vi "Swerve Controller.vi"(8 "error in":errorcluster) -> ()   [LabVIEW 2023]
doc: "This VI executes continuously carrying out the current operation and responding to updates or new operations. It will often contain the timing or control code that is difficult to place directly in TeleOp. This VI generally opens all sensors and motors and isolates the rest of the robot code from knowing how the operations are carried out."
uses:
  <vilib>/Rock Robotics/WPI/Framework/Completion Status.ctl
  Swerve Setpoints2.ctl
  Swerve Operations.ctl
  Framework/Robot Global Data.vi
  <vilib>/addons/control/pid/pid.llb/PID (DBL).vi
  <vilib>/addons/control/pid/NI_PID_pid.lvlib
  <vilib>/Rock Robotics/Network Tables/NT Write Boolean.vi
panel:
  out "error out":errorcluster
  out "x-y":u32
  in  "Tape":T1={"proportional gain (Kc)"=1.0, "integral time (Ti, min)"=0.01, "derivative time (Td, min)"=0.0} {"derivative time (Td, min)" format="%.3f"; "integral time (Ti, min)" format="%.3f"; "proportional gain (Kc)" format="%.3f"}
  in  "AprilTag":T1={"proportional gain (Kc)"=1.0, "integral time (Ti, min)"=0.01, "derivative time (Td, min)"=0.0} {"derivative time (Td, min)" format="%.3f"; "integral time (Ti, min)" format="%.3f"; "proportional gain (Kc)" format="%.3f"}
  in  "Look At Cube":T1={"proportional gain (Kc)"=0.001, "integral time (Ti, min)"=0.0, "derivative time (Td, min)"=0.0}
  in  "Look At Cone":T1={"proportional gain (Kc)"=0.004, "integral time (Ti, min)"=0.0, "derivative time (Td, min)"=0.01}
  in  "Balance":T1={"proportional gain (Kc)"=0.011, "integral time (Ti, min)"=0.0, "derivative time (Td, min)"=0.0} {"derivative time (Td, min)" format="%.3f"; "integral time (Ti, min)" format="%.3f"; "proportional gain (Kc)" format="%.3f"}
  in  "Drive to Angle(Distance)":T1={"proportional gain (Kc)"=0.9, "integral time (Ti, min)"=0.0, "derivative time (Td, min)"=0.0} {"derivative time (Td, min)" format="%.3f"; "integral time (Ti, min)" format="%.3f"; "proportional gain (Kc)" format="%.3f"}
  in  "Drive to Angle(Distance)":T1={"proportional gain (Kc)"=0.022, "integral time (Ti, min)"=0.0, "derivative time (Td, min)"=0.0} {"derivative time (Td, min)" format="%.3f"; "integral time (Ti, min)" format="%.3f"; "proportional gain (Kc)" format="%.3f"}
  out "Gyro":dbl
  in  "Drive to angle(Time)":T1={"proportional gain (Kc)"=0.019999999999999574, "integral time (Ti, min)"=0.0, "derivative time (Td, min)"=0.0} {"derivative time (Td, min)" format="%.3f"; "integral time (Ti, min)" format="%.3f"; "proportional gain (Kc)" format="%.3f"}
  in  "Turn to Angle":T1={"proportional gain (Kc)"=0.019999999999999574, "integral time (Ti, min)"=0.0, "derivative time (Td, min)"=0.0} {"derivative time (Td, min)" format="%.3f"; "integral time (Ti, min)" format="%.3f"; "proportional gain (Kc)" format="%.3f"}
  in  "Interactive Values":T2
  out "Current\nCmd":string="Started at  16:27:40.452\nDefault: Reserve,  S 0.0, D 0.000000"
  in  "Buttons":cluster{"Execute Cmd":bool, "Abort Cmd":bool}
  out "Command Timing":cluster{"Start Time (ms)":u32, "Iterations":i32}={"Start Time (ms)"=1585114, "Iterations"=-1}
  out "Status":T4=enum."Aborted"
  # "Tip: It may be helpful to observe inputs and sensor values.\nYou may also want to display tuning or debugging controls."
  # "Interactive Command: You may fill in the settings for a command\nand schedule it with the Execute button. You can observe and abort\nany command while fine tuning the code for the controller."
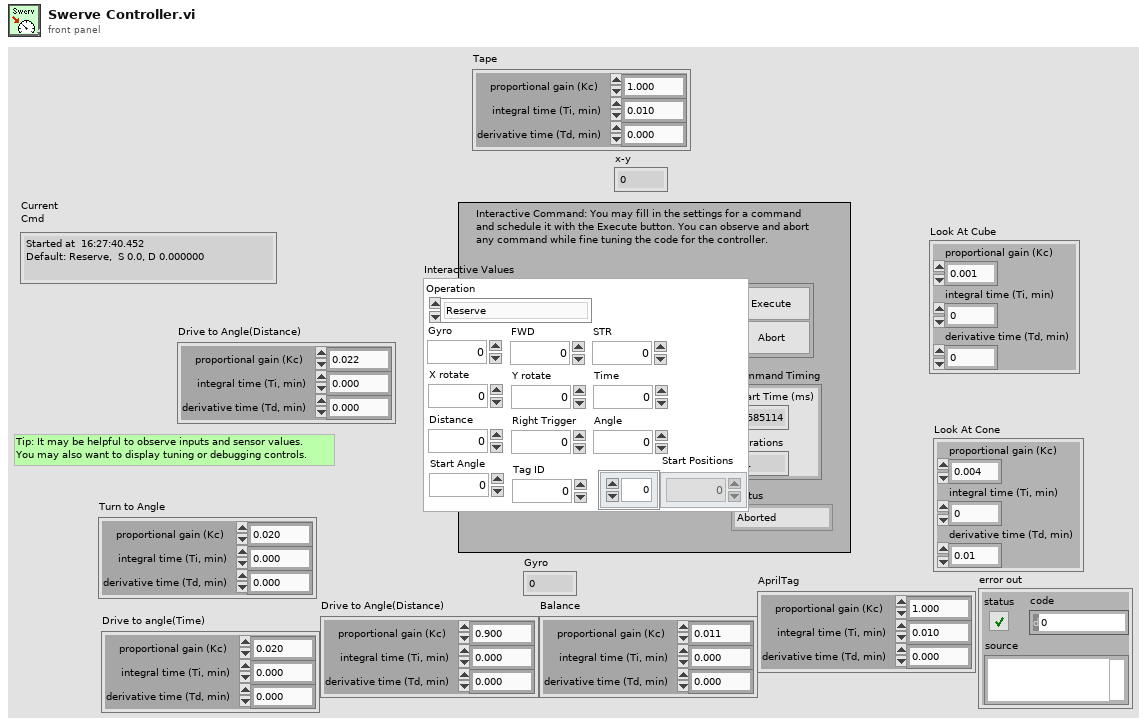
[diagram p1: front panel]
types:
  T1 = cluster{"proportional gain (Kc)":dbl, "integral time (Ti, min)":dbl, "derivative time (Td, min)":dbl}
  T2 = typedef "Swerve Setpoints2.ctl" = cluster{"Operation":T3, "Gyro":dbl, "FWD":dbl, "STR":dbl, "X rotate":dbl, "Y rotate":dbl, "Time":dbl, "Distance":dbl, "Right Trigger":dbl, "Angle":dbl, "Start Angle":dbl, "Tag ID":dbl, "Start Positions":dbl[]}
  T3 = typedef "Swerve Operations.ctl" = enum16{"Reserve", "Read Current", "Immediate", "Stop", "Balance", "Direct  Joystick Drive", "Joystick Drive", "Drive for Distance", "Drive for Time", "Turn to Angle", "Drive to Angle(Time)", "Drive to Angle(Distance)", "Look At Cone", "Look At Cube", "Move To Tape", "Move To Tag"}
  T4 = typedef "Completion Status.ctl" = enum16{"Successful", "Aborted", "Incomplete"}
  T5 = typedef "Command Status Info.ctl" = cluster{"Name":string, "Status":T4, "notifier out":T6}
  T6 = typedef "Completion Notifier.ctl" = refnum<notifier>
  T7 = cluster{"Current Command":T2, "Command Timing":cluster{"Start Time (ms)":u32, "Iterations":i32}, "Command Arguments":cluster{"Command Info":T5, "Description":string, "Default Command":T2, "queue out":refnum<queue>, "Subsystem Name":string}}
  T8 = enum16{"AprilTag", "Reflective Tape", "Custom", "Cube", "Cone"}
  T9 = typedef "ADIS16470 Device Reference.ctl" = cluster{"DevStatus":errorcluster, "Hardware Config":T10, "Calibration Complete":refnum<notifier>, "Status Reference":refnum<data-value>, "Data Reference":refnum<data-value>, "Sychronous Process VI":T14, "Cmd FIFO":refnum<k33>, "Source":T15, "Data FIFO":refnum<k33>, "Calibration Time (ms)":u32, "Data Reference":refnum<data-value>}
  T10 = typedef "ADIS16470 Hardware Configuration.ctl" = cluster{"SPI Clock Rate (Hz)":dbl, "IMU SPI Mode (3)":T11, "IMU Reset Pin":T12, "IMU SPI Bus":T13, "IMU Data Ready Pin":T12, "Stall Config":cluster{"Pow2BytesPerRead":u8, "StallTicks":u16, "CsToSclkTicks":u8}}
  T11 = typedef "WPI_SPIMode.ctl" = enum16{"Mode 0 (Clk Idle Low,Sample on Leading)", "Mode 1 (Clk Idle Low,Sample on Trailing)", "Mode 2 (Clk Idle High,Sample on Leading)", "Mode 3 (Clk Idle High,Sample on Trailing)"}
  T12 = typedef "FPGA_DIOChannel.ctl" = enum8{"DIO 0", "DIO 1", "DIO 2", "DIO 3", "DIO 4", "DIO 5", "DIO 6", "DIO 7", "DIO 8", "DIO 9", "DIO MXP 0", "DIO MXP 1", "DIO MXP 2", "DIO MXP 3", "DIO MXP 4", "DIO MXP 5", "DIO MXP 6", "DIO MXP 7", "DIO MXP 8", "DIO MXP 9", "DIO MXP 10", "DIO MXP 11", "DIO MXP 12", "DIO MXP 13", "DIO MXP 14", "DIO MXP 15", "SPI Port CS1", "SPI Port CS2", "SPI Port CS3", "SPI Port MISO", "SPI Port MOSI", "Invalid"}
  T13 = typedef "spi_bus.ctl" = enum16{"SPI On-Board, CS0", "SPI On-Board, CS1", "SPI On-Board, CS2", "SPI On-Board, CS3", "SPI MXP", "Invalid"}
  T14 = typedef "ADIS16470 Process.ctl" = refnum<vi>
  T15 = typedef "FPGA_CounterEncoderSourceConvertionLVSourceType.ctl" = cluster{"DevStatus":errorcluster, "AnalogTriggerMode?":bool, "DigitalMode":cluster{"DIO Channel":T16}, "AnalogTriggerMode":cluster{"AnalogTriggerIndex":T17, "OutputType":T18}}
  T16 = typedef "FPGA_DIODigitalSourceChannel.ctl" = enum8{"DIO 0", "DIO 1", "DIO 2", "DIO 3", "DIO 4", "DIO 5", "DIO 6", "DIO 7", "DIO 8", "DIO 9", "DIO MXP 0", "DIO MXP 1", "DIO MXP 2", "DIO MXP 3", "DIO MXP 4", "DIO MXP 5", "DIO MXP 6", "DIO MXP 7", "DIO MXP 8", "DIO MXP 9", "DIO MXP 10", "DIO MXP 11", "DIO MXP 12", "DIO MXP 13", "DIO MXP 14", "DIO MXP 15", "SPI Port CS1", "SPI Port CS2", "SPI Port CS3", "SPI Port MISO", "SPI Port MOSI", "Disabled"}
  T17 = typedef "FPGA_AnalogTriggerIndex.ctl" = enum8{"Trig 0", "Trig 1", "Trig 2", "Trig 3", "Trig 4", "Trig 5", "Trig 6", "Trig 7", "Invalid"}
  T18 = typedef "FPGA_AnalogTriggerOutType.ctl" = enum16{"InWindow", "TriggerState", "Rising", "Falling"}
  T19 = typedef "ADIS16470 Data.ctl" = cluster{"XAngle":dbl, "YAngle":dbl, "ZAngle":dbl}
  T20 = typedef "WPI_MotorControlDeviceRef.ctl" = cluster{"DeviceStatus":errorcluster, "Type":T21, "PWM":cluster{"PWM Channel":T22, "DeadBand":T23}, "CAN":cluster{"Device Number":u8, "SetOutput VI Ref":variant, "GetOutput VI Ref":variant, "Enable VI Ref":variant, "Disable VI Ref":variant, "Data":variant}, "Invert":bool, "DIO PWM":cluster{"PWM \"Enable\" Channel":T22, "DIOChannel":T12, "PWM Rate":dbl}}
  T21 = typedef "WPI_MotorControlType.ctl" = enum16{"PWM", "CAN", "DIO PWM"}
  T22 = typedef "FPGA_DIOPWMChannel.ctl" = enum8{"PWM 0", "PWM 1", "PWM 2", "PWM 3", "PWM 4", "PWM 5", "PWM 6", "PWM 7", "PWM 8", "PWM 9", "PWM MXP 0", "PWM MXP 1", "PWM MXP 2", "PWM MXP 3", "PWM MXP 4", "PWM MXP 5", "PWM MXP 6", "PWM MXP 7", "PWM MXP 8", "PWM MXP 9", "Invalid"}
  T23 = typedef "WPI_PWMDeadband.ctl" = cluster{"Name":string, "maxPositivePwm":i32, "minPositivePwm":i32, "centerPwm":i32, "maxNegativePwm":i32, "minNegativePwm":i32, "angularRange":u16}
  T24 = cluster{"tag ID":i32, "Center":cluster{"X":dbl, "Y":dbl}, "homography matrix":dbl[], "decision margin":dbl, "Hamming Dist":i32, "corner points":cluster{"X":dbl, "Y":dbl}[], "Tag Family":string}[]
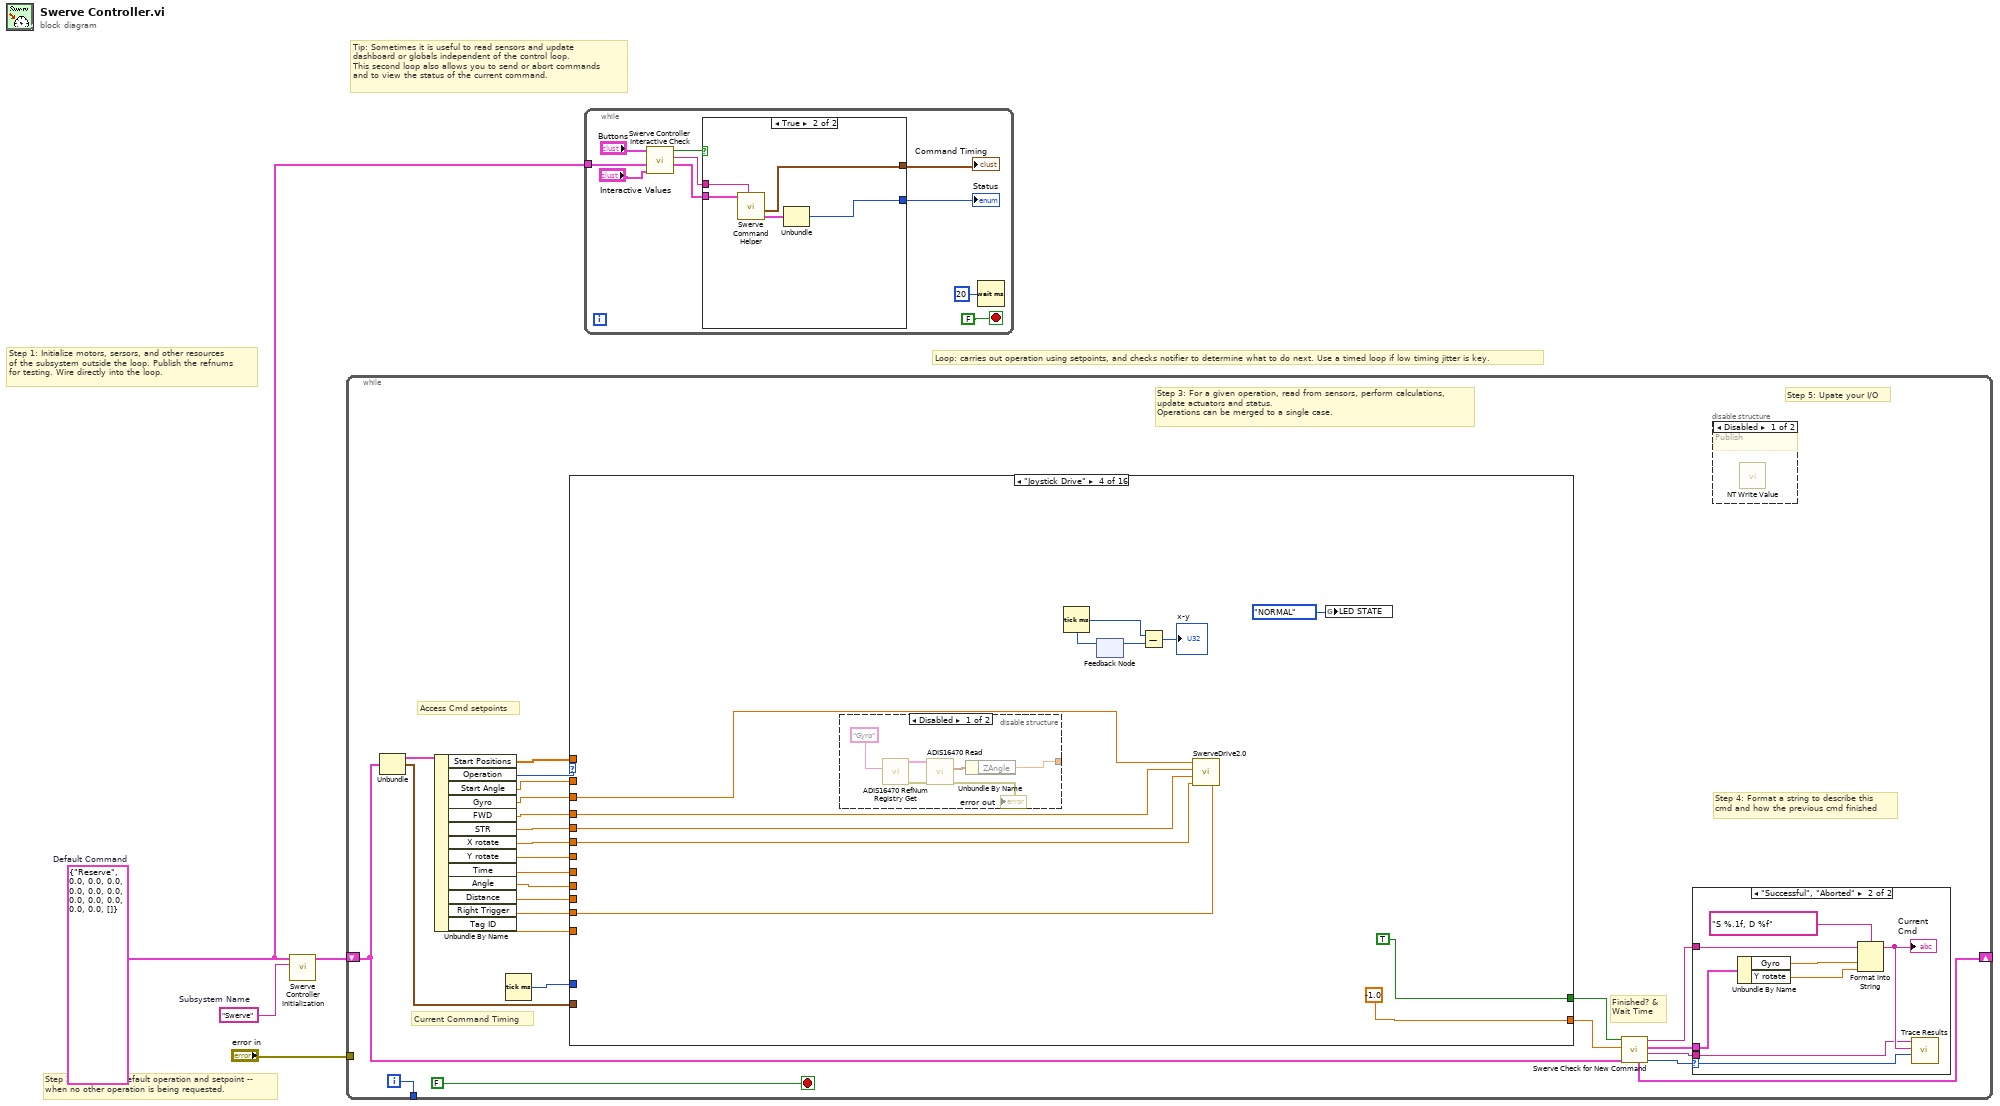
[diagram p0: block diagram]
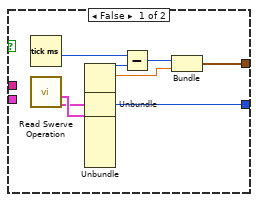
[diagram p2: hidden frame]
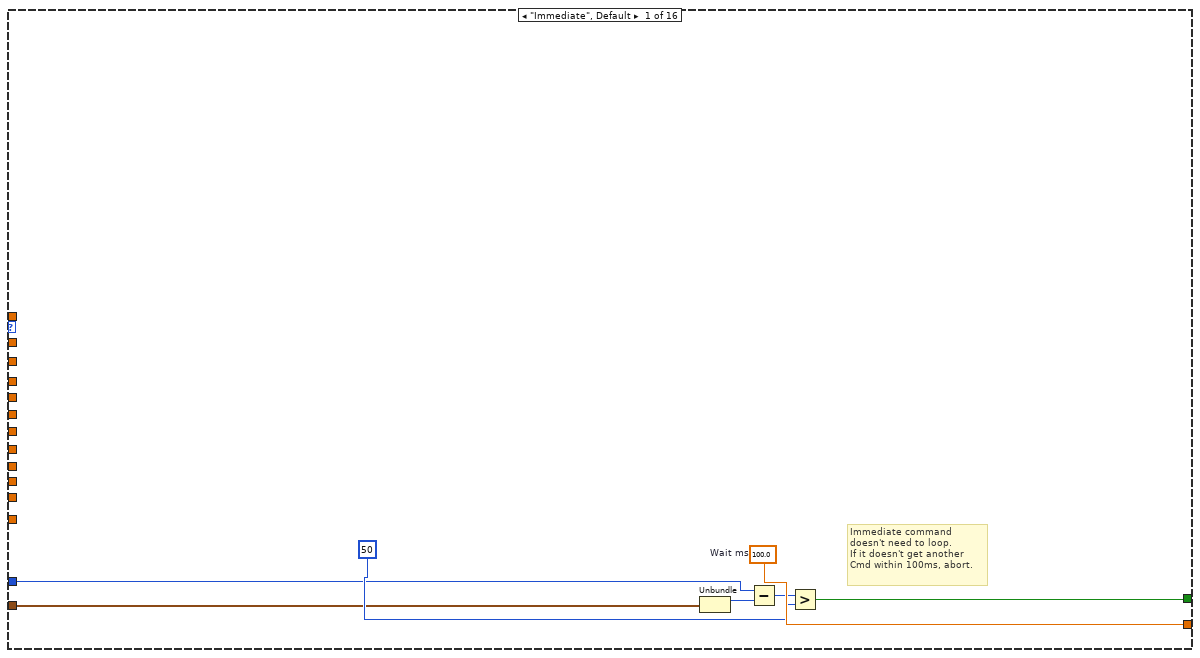
[diagram p3: hidden frame]
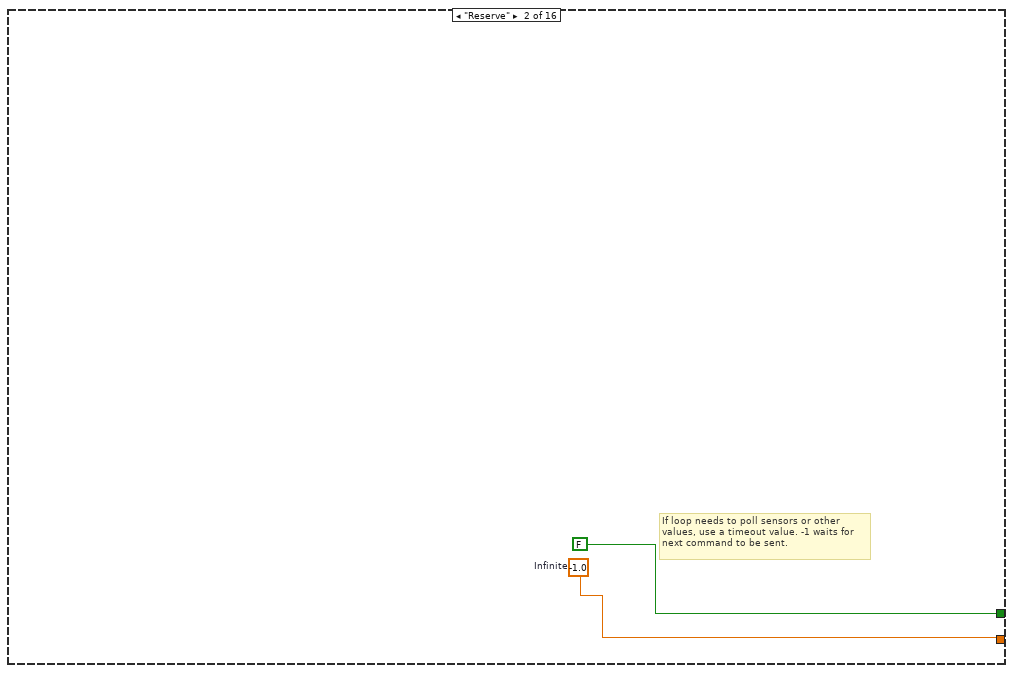
[diagram p4: hidden frame]
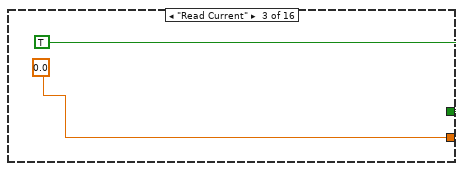
[diagram p5: hidden frame]
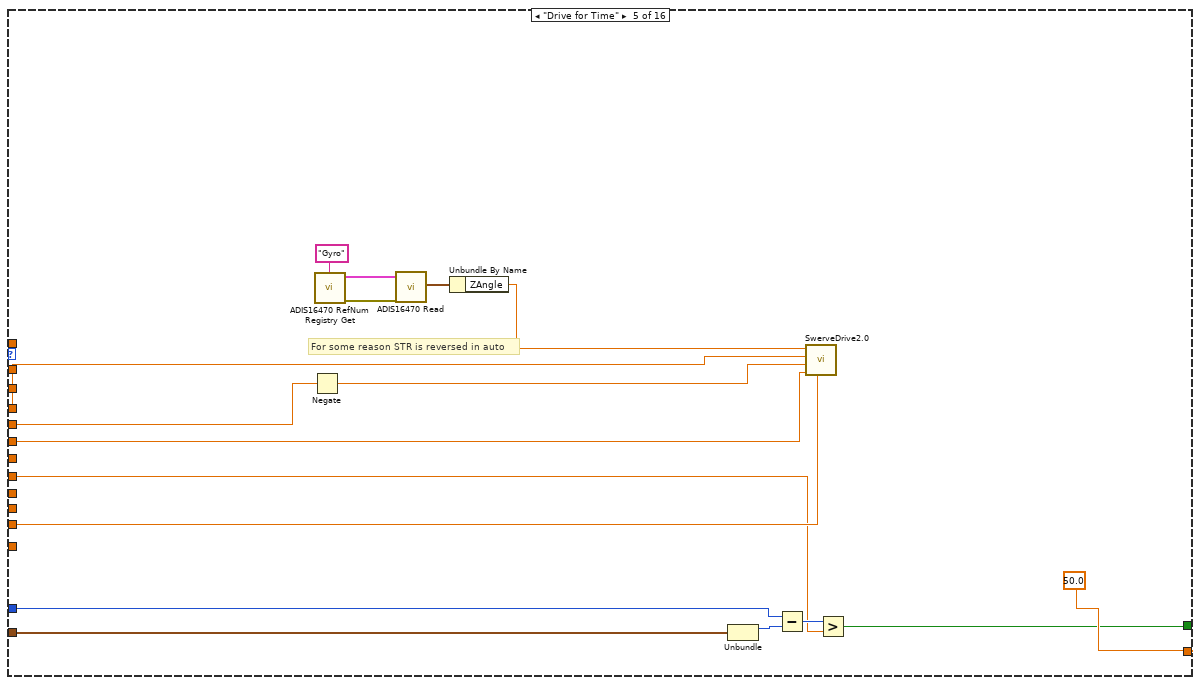
[diagram p7: hidden frame]
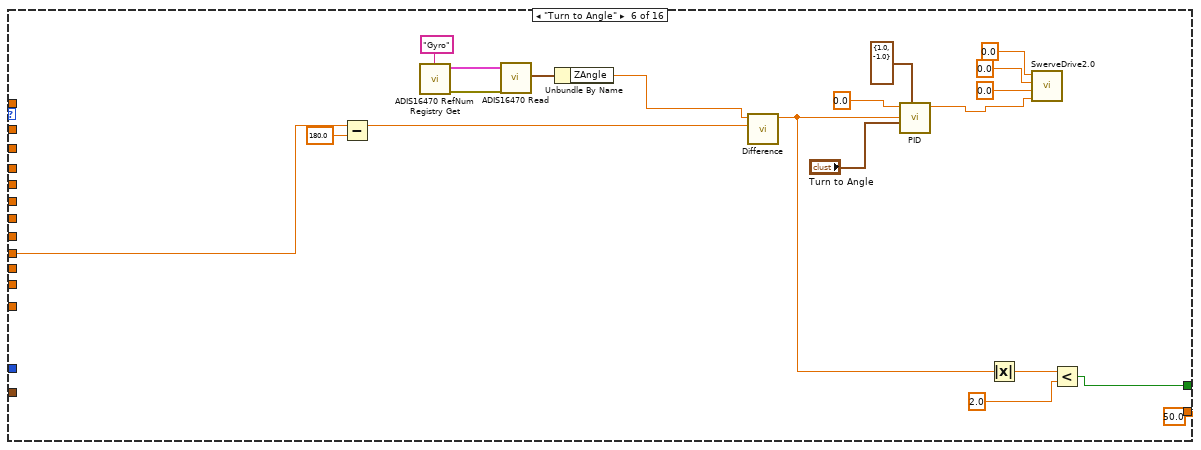
[diagram p8: hidden frame]
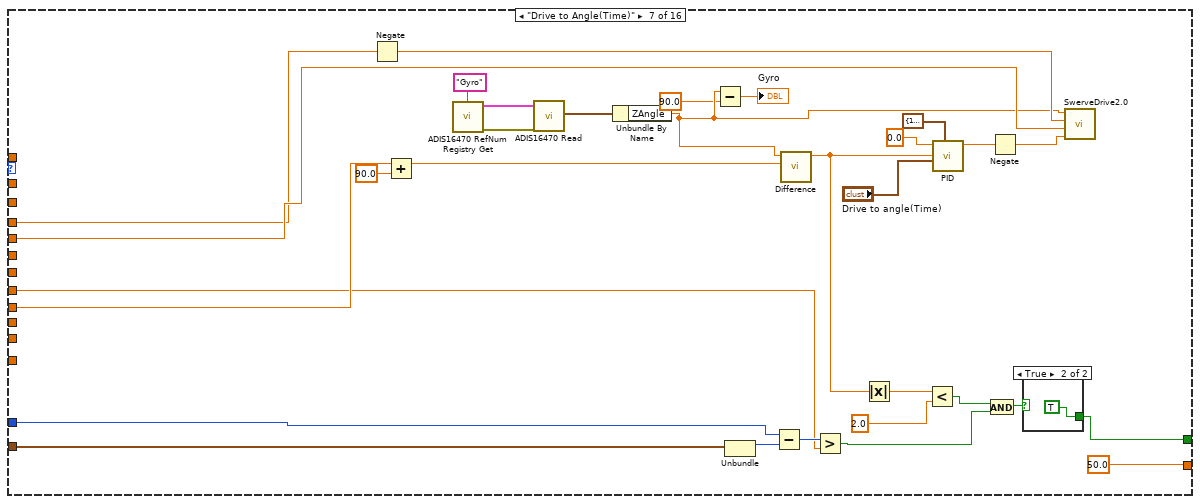
[diagram p9: hidden frame]
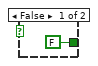
[diagram p10: hidden frame]
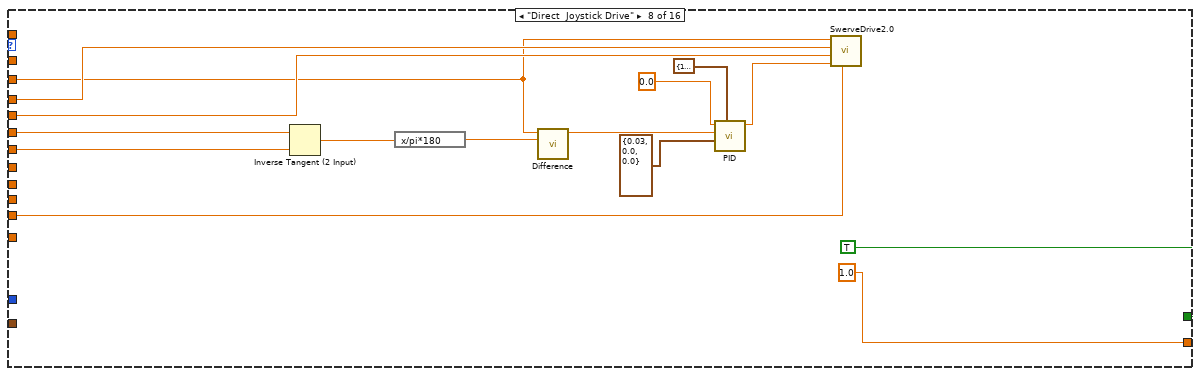
[diagram p11: hidden frame]
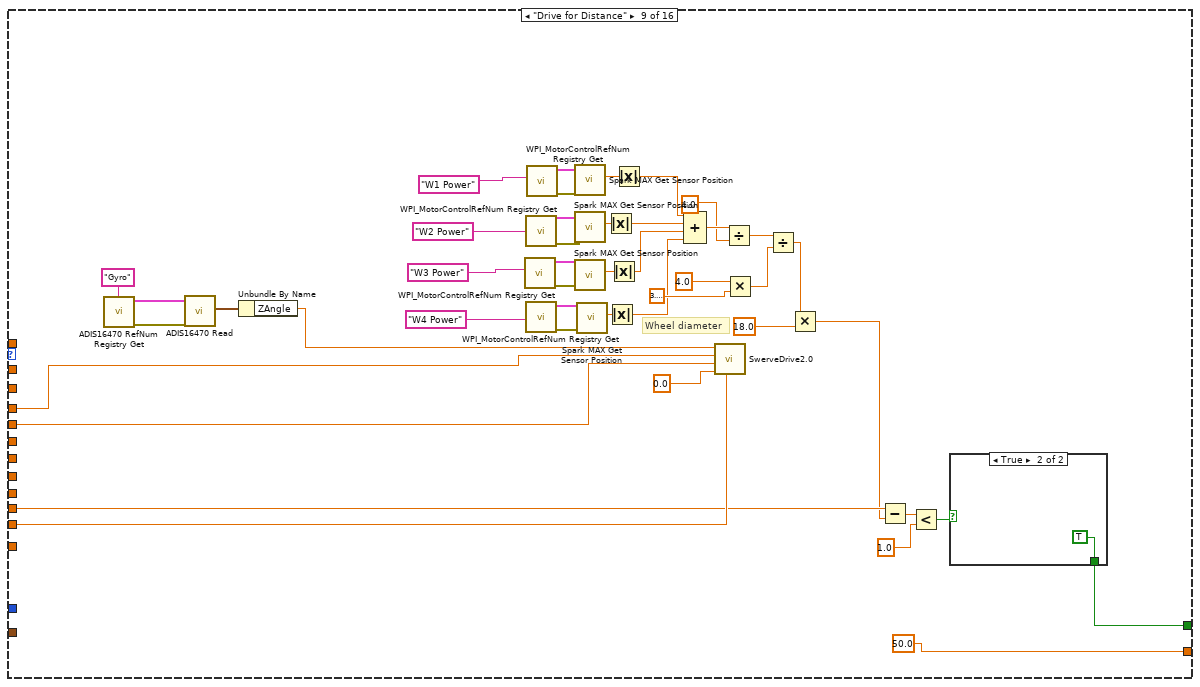
[diagram p12: hidden frame]
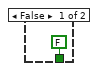
[diagram p13: hidden frame]
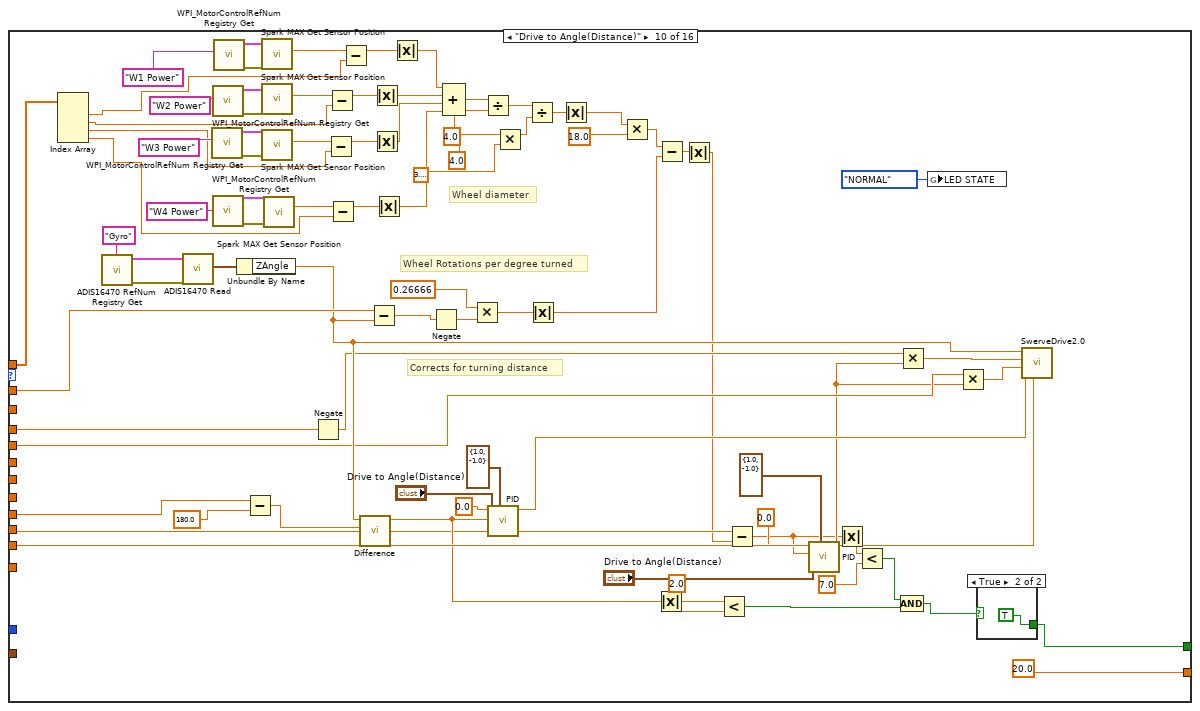
[diagram p14: hidden frame]
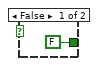
[diagram p15: hidden frame]
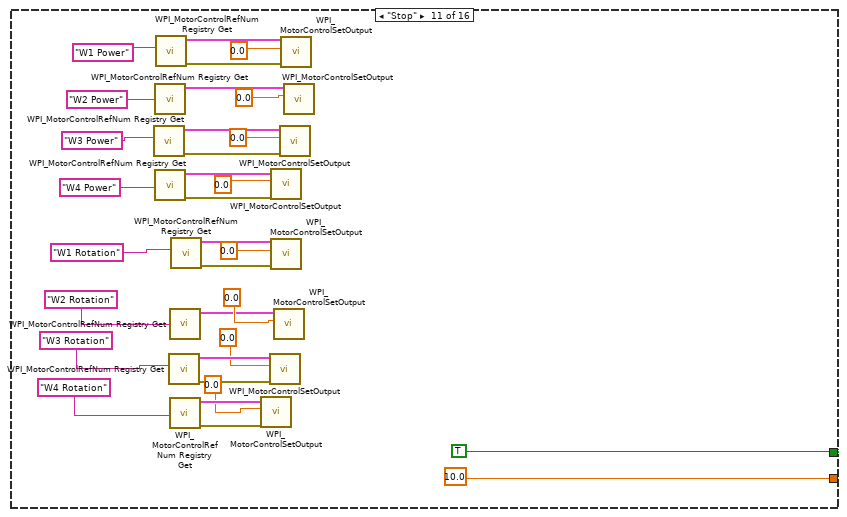
[diagram p16: hidden frame]
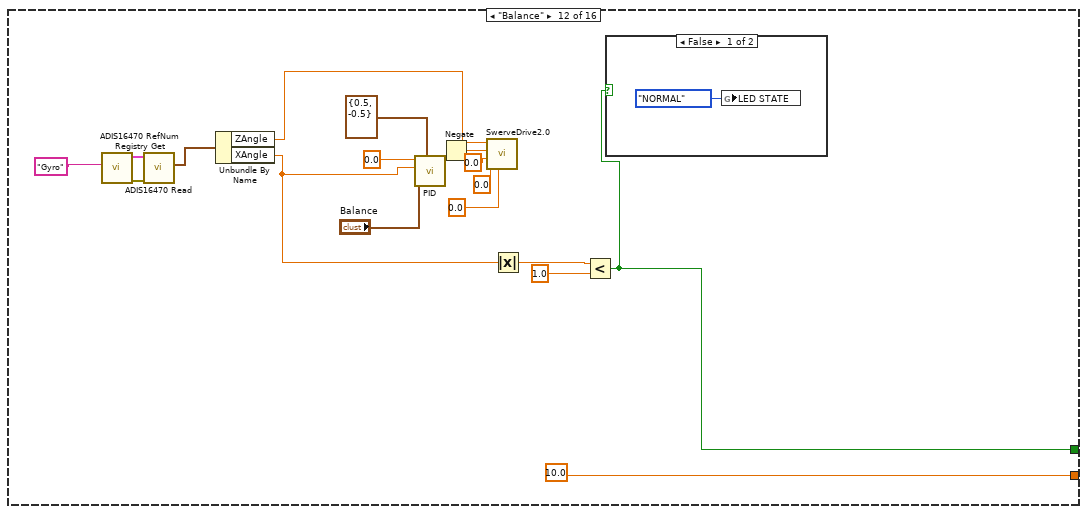
[diagram p17: hidden frame]
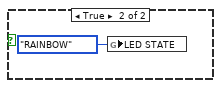
[diagram p18: hidden frame]
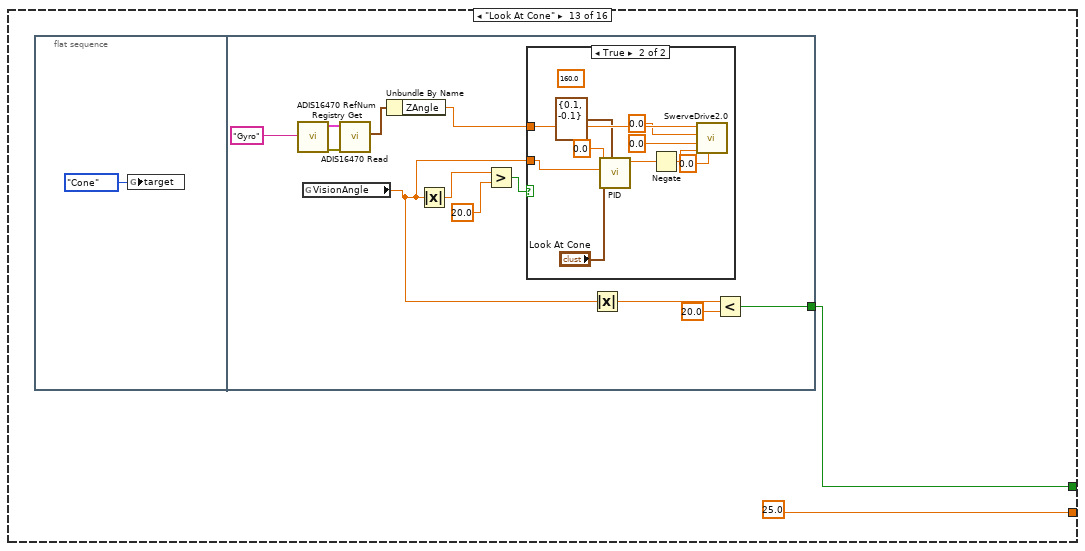
[diagram p19: hidden frame]
diagram:
  w1 = T2 {"Operation"=enum."Reserve", "Gyro"=0.0, "FWD"=0.0, "STR"=0.0, "X rotate"=0.0, "Y rotate"=0.0, "Time"=0.0, "Distance"=0.0, "Right Trigger"=0.0, "Angle"=0.0, "Start Angle"=0.0, "Tag ID"=0.0, "Start Positions"=[]}  # Default Command
  w2 = "Swerve"  # Subsystem Name
  # "Tip: Sometimes it is useful to read sensors and update\ndashboard or globals independent of the control loop.\nThis second loop also allows you to send or abort commands\nand to view the status of the current command."
  # "Step 2: Define the default operation and setpoint --\nwhen no other operation is being requested."
  # "Step 1: Initialize motors, sersors, and other resources\nof the subsystem outside the loop. Publish the refnums\nfor testing. Wire directly into the loop."
  # "Loop: carries out operation using setpoints, and checks notifier to determine what to do next. Use a timed loop if low timing jitter is key."
  n1 = call "Swerve Controller Initialization.vi"("Subsystem Name"=w2, "Default Command"=w1) -> ("Current Command"=w3:T7)  [unwired: 9 in]
  n2 = while {
    shift-right: [w24] -> _
    shift-left: w3 -> [w18]
    tunnel: [w29] -> _
    tunnel: "error in" -> [_]
    i -> [w29]
    stop <- FALSE stop-if-true
    # "Step 5: Upate your I/O"
    # "Step 4: Format a string to describe this\ncmd and how the previous cmd finished"
    # "Current Command Timing"
    # "Access Cmd setpoints"
    # "Finished? &\nWait Time"
    # "Step 3: For a given operation, read from sensors, perform calculations,\nupdate actuators and status.\nOperations can be merged to a single case."
    n3 = Unbundle(w18) -> ("Current Command"=w28:T2, "Command Timing"=w25:cluster{"Start Time (ms)":u32, "Iterations":i32})  [unwired: 1 out]
    n4 = Unbundle By Name(w28) -> ("Start Positions"=w5:dbl[], "Operation"=w27:T3, "Start Angle"=w8:dbl, "Gyro"=w17:dbl, "FWD"=w16:dbl, "STR"=w15:dbl, "X rotate"=w14:dbl, "Y rotate"=w9:dbl, "Time"=w10:dbl, "Angle"=w13:dbl, "Distance"=w12:dbl, "Right Trigger"=w11:dbl, "Tag ID"=w7:dbl)
    n5 = Tick Count (ms)() -> (millisecond timer value=w26:u32)
    n6 = case shown="\"Joystick Drive\"" w27 {
      tunnel: [w37 w39 0.0 ("Time") -1.0 ("Infinite") 50.0 ("Time") 50.0 ("Time") 50.0 ("Time") 1.0 ("Time") 50.0 ("Time") 20.0 ("Time") 10.0 ("Time") 10.0 ("Time") 25.0 ("Time") 25.0 ("Time") 10.0 ("Time") 10.0 ("Time")] -> w23
      tunnel: w25 -> [w33 _ _ _ w69 _ w124 _ _ _ _ _ _ _ _ _]
      tunnel: w26 -> [w32 _ _ _ w70 _ w123 _ _ _ _ _ _ _ _ _]
      tunnel: w17 -> [_ _ _ w42 _ _ _ w130 _ _ _ _ _ _ _ _]
      tunnel: w16 -> [_ _ _ w52 w73 _ w103 w141 w145 w268 _ _ _ _ _ _]
      tunnel: w15 -> [_ _ _ w49 w74 _ w104 w142 w167 w205 _ _ _ _ _ _]
      tunnel: w14 -> [_ _ _ w48 w66 _ _ w136 _ _ _ _ _ _ _ _]
      tunnel: w13 -> [_ _ _ _ _ w80 w102 _ _ w267 _ _ _ _ _ _]
      tunnel: w12 -> [_ _ _ _ _ _ _ _ w165 w221 _ _ _ _ _ _]
      tunnel: w11 -> [_ _ _ w51 w75 _ _ w143 w187 w269 _ _ _ _ _ _]
      tunnel: w10 -> [_ _ _ _ w67 _ w101 _ _ _ _ _ _ _ _ _]
      tunnel: w9 -> [_ _ _ _ _ _ _ w135 _ _ _ _ _ _ _ _]
      tunnel: w8 -> [_ _ _ _ _ _ _ _ _ w217 _ _ _ _ _ _]
      tunnel: w7 -> [_ _ _ _ _ _ _ _ _ _ _ _ _ _ w380 _]
      tunnel: [w31 FALSE ("ignore previous (F)") TRUE ("ignore previous (F)") TRUE ("ignore previous (F)") w59 w76 w96 TRUE ("ignore previous (F)") w144 w203 TRUE ("ignore previous (F)") w306 w326 w351 w379 w415] -> w6
      tunnel: w5 -> [_ _ _ _ _ _ _ _ _ w196 _ _ _ _ _ _]
      frame "Immediate", Default {
        w37 = 100.0  # Wait ms
        # "Immediate command\ndoesn't need to loop.\nIf it doesn't get another\nCmd within 100ms, abort."
        n7 = Unbundle(w33) -> ("Start Time (ms)"=w36:u32)  [unwired: 1 out]
        n8 = Subtract(x=w32, y=w36) -> (x-y=w35:u32)
        n9 = Greater?(x=w35, y=u8 50 ("Left Motor")) -> (0:w31:bool)
      }
      frame "Reserve" {
        w39 = -1.0  # Infinite
        # "If loop needs to poll sensors or other\nvalues, use a timeout value. -1 waits for\nnext command to be sent."
      }
      frame "Read Current" {
      }
      frame "Joystick Drive" {
        n10 = disable-structure shown="Disabled" {
          disable-tunnel: [w54 _] -> _
          frame Disabled {
            n11 = call <vilib>:"ADIS16470 RefNum Registry Get.vi"("refnum name"="Gyro") -> ("error out"=w58:errorcluster, "ADIS16470DevRef out"=w57:T9)  [unwired: 9 in]
            n12 = call <vilib>:"ADIS16470 Read.vi"("error in (no error)"=w58, "ADIS16470DevRef"=w57) -> ("error out"=→"error out":errorcluster, "ADIS16470 Value"=w55:T19)  [unwired: 6 in, 2 out]
            n13 = Unbundle By Name(w55) -> ("ZAngle"=w54:dbl)
          }
          frame Enabled {
          }
        }
        n14 = Tick Count (ms)() -> (millisecond timer value=w46:u32)
        n15 = feedback-in #1(w46) -> ()
        n16 = feedback #1() -> (w45:u32)  [unwired: 1 in]
        n17 = Subtract(x=w46, y=w45) -> (x-y=→"x-y":u32)
        n18 = call "SwerveDrive2.0.vi"("Right Trigger"=w51, "RCW"=w48, "STR"=w49, "FWD"=w52, "Gyro"=w42) -> ()  [unwired: 7 in]
        n19 = global write "Robot Global Data.vi" "LED STATE"(enum16{"NORMAL", "RAINBOW"}."NORMAL" ("LED STATE")) -> ()
      }
      frame "Drive for Time" {
        # "For some reason STR is reversed in auto"
        n20 = Negate(x=w74) -> (-x=w60:dbl)
        n21 = call <vilib>:"ADIS16470 RefNum Registry Get.vi"("refnum name"="Gyro") -> ("error out"=w65:errorcluster, "ADIS16470DevRef out"=w64:T9)  [unwired: 9 in]
        n22 = call <vilib>:"ADIS16470 Read.vi"("error in (no error)"=w65, "ADIS16470DevRef"=w64) -> ("ADIS16470 Value"=w63:T19)  [unwired: 6 in, 3 out]
        n23 = Unbundle By Name(w63) -> ("ZAngle"=w61:dbl)
        n24 = Unbundle(w69) -> ("Start Time (ms)"=w72:u32)  [unwired: 1 out]
        n25 = Subtract(x=w70, y=w72) -> (x-y=w71:u32)
        n26 = call "SwerveDrive2.0.vi"("Right Trigger"=w75, "RCW"=w66, "STR"=w60, "FWD"=w73, "Gyro"=w61) -> ()  [unwired: 7 in]
        n27 = Greater?(x=w71, y=w67) -> (0:w59:bool)
      }
      frame "Turn to Angle" {
        n28 = Subtract(x=w80, y=180.0) -> (x-y=w79:dbl)
        n29 = call <vilib>:"ADIS16470 RefNum Registry Get.vi"("refnum name"="Gyro") -> ("error out"=w90:errorcluster, "ADIS16470DevRef out"=w89:T9)  [unwired: 9 in]
        n30 = call <vilib>:"ADIS16470 Read.vi"("error in (no error)"=w90, "ADIS16470DevRef"=w89) -> ("ADIS16470 Value"=w88:T19)  [unwired: 6 in, 3 out]
        n31 = Unbundle By Name(w88) -> ("ZAngle"=w86:dbl)
        n32 = call "Difference.vi"("Angle"=w79, "Gyro"=w86) -> ("Difference"=w84:dbl)  [unwired: 9 in]
        n33 = call-poly <vilib>:"PID.vi"("output range"=cluster{"output high":dbl, "output low":dbl} {"output high"=1.0, "output low"=-1.0}, "PID gains"="Turn to Angle", "process variable"=w84, "setpoint"=0.0) -> ("output"=w77:dbl)  [unwired: 6 in, 1 out]
        n34 = Absolute Value(x=w84) -> (abs(x)=w82:dbl)
        n35 = call "SwerveDrive2.0.vi"("RCW"=w77, "STR"=0.0, "FWD"=0.0, "Gyro"=0.0) -> ()  [unwired: 8 in]
        n36 = Less?(x=w82, y=2.0) -> (x < y?=w76:bool)
      }
      frame "Drive to Angle(Time)" {
        n37 = Negate(x=w103) -> (-x=w100:dbl)
        n38 = Add(x=w102, y=90.0) -> (x+y=w111:dbl)
        n39 = call <vilib>:"ADIS16470 RefNum Registry Get.vi"("refnum name"="Gyro") -> ("error out"=w116:errorcluster, "ADIS16470DevRef out"=w115:T9)  [unwired: 9 in]
        n40 = call <vilib>:"ADIS16470 Read.vi"("error in (no error)"=w116, "ADIS16470DevRef"=w115) -> ("ADIS16470 Value"=w114:T19)  [unwired: 6 in, 3 out]
        n41 = Unbundle By Name(w114) -> ("ZAngle"=w99:dbl)
        n42 = Subtract(x=w99, y=90.0) -> (x-y=→"Gyro":dbl)
        n43 = Unbundle(w124) -> ("Start Time (ms)"=w126:u32)  [unwired: 1 out]
        n44 = Subtract(x=w123, y=w126) -> (x-y=w125:u32)
        n45 = call "Difference.vi"("Angle"=w111, "Gyro"=w99) -> ("Difference"=w108:dbl)  [unwired: 9 in]
        n46 = Greater?(x=w125, y=w101) -> (0:w121:bool)
        n47 = Absolute Value(x=w108) -> (abs(x)=w106:dbl)
        n48 = Less?(x=w106, y=2.0) -> (x < y?=w105:bool)
        n49 = call-poly <vilib>:"PID.vi"("output range"=cluster{"output high":dbl, "output low":dbl} {"output high"=1.0, "output low"=-1.0}, "PID gains"="Drive to angle(Time)", "process variable"=w108, "setpoint"=0.0) -> ("output"=w117:dbl)  [unwired: 6 in, 1 out]
        n50 = And(x=w105, y=w121) -> (x .and. y?=w122:bool)
        n51 = Negate(x=w117) -> (-x=w109:dbl)
        n52 = case shown="True" w122 {
          tunnel: [FALSE ("ignore previous (F)") TRUE ("ignore previous (F)")] -> w96
          frame False {
          }
          frame True {
          }
        }
        n53 = call "SwerveDrive2.0.vi"("RCW"=w109, "STR"=w104, "FWD"=w100, "Gyro"=w99) -> ()  [unwired: 8 in]
      }
      frame "Direct  Joystick Drive" {
        n54 = Inverse Tangent (2 Input)(1:w135, 2:w136) -> (0:w133:dbl)
        n55 = expression code="x/pi*180"(w133) -> (w131:dbl)
        n56 = call "Difference.vi"("Angle"=w131, "Gyro"=w130) -> ("Difference"=w132:dbl)  [unwired: 9 in]
        n57 = call-poly <vilib>:"PID.vi"("output range"=cluster{"output high":dbl, "output low":dbl} {"output high"=1.0, "output low"=-1.0}, "PID gains"=T1 {"proportional gain (Kc)"=0.03, "integral time (Ti, min)"=0.0, "derivative time (Td, min)"=0.0}, "process variable"=w132, "setpoint"=0.0) -> ("output"=w140:dbl)  [unwired: 6 in, 1 out]
        n58 = call "SwerveDrive2.0.vi"("Right Trigger"=w143, "RCW"=w140, "STR"=w142, "FWD"=w141, "Gyro"=w130) -> ()  [unwired: 7 in]
      }
      frame "Drive for Distance" {
        # "Wheel diameter"
        n59 = call <vilib>:"ADIS16470 RefNum Registry Get.vi"("refnum name"="Gyro") -> ("error out"=w162:errorcluster, "ADIS16470DevRef out"=w161:T9)  [unwired: 9 in]
        n60 = call <vilib>:"ADIS16470 Read.vi"("error in (no error)"=w162, "ADIS16470DevRef"=w161) -> ("ADIS16470 Value"=w160:T19)  [unwired: 6 in, 3 out]
        n61 = Unbundle By Name(w160) -> ("ZAngle"=w158:dbl)
        n62 = call <vilib>:"WPI_MotorControlRefNum Registry Get.vi"("refnum name"="W3 Power") -> ("error out"=w181:errorcluster, "MotorControlDevRef"=w180:T20)  [unwired: 9 in]
        n63 = call <vilib>:"WPI_MotorControlRefNum Registry Get.vi"("refnum name"="W2 Power") -> ("error out"=w183:errorcluster, "MotorControlDevRef"=w182:T20)  [unwired: 9 in]
        n64 = call <vilib>:"WPI_MotorControlRefNum Registry Get.vi"("refnum name"="W4 Power") -> ("error out"=w179:errorcluster, "MotorControlDevRef"=w178:T20)  [unwired: 9 in]
        n65 = call <vilib>:"WPI_MotorControlRefNum Registry Get.vi"("refnum name"="W1 Power") -> ("error out"=w185:errorcluster, "MotorControlDevRef"=w184:T20)  [unwired: 9 in]
        n66 = call <vilib>:"Spark MAX Get Sensor Position.vi"("error in (no error)"=w185, "MotorControlDevRef in"=w184) -> ("Sensor Position"=w170:dbl)  [unwired: 6 in, 3 out]
        n67 = call <vilib>:"Spark MAX Get Sensor Position.vi"("error in (no error)"=w183, "MotorControlDevRef in"=w182) -> ("Sensor Position"=w171:dbl)  [unwired: 6 in, 3 out]
        n68 = call <vilib>:"Spark MAX Get Sensor Position.vi"("error in (no error)"=w181, "MotorControlDevRef in"=w180) -> ("Sensor Position"=w172:dbl)  [unwired: 6 in, 3 out]
        n69 = call <vilib>:"Spark MAX Get Sensor Position.vi"("error in (no error)"=w179, "MotorControlDevRef in"=w178) -> ("Sensor Position"=w173:dbl)  [unwired: 6 in, 3 out]
        n70 = Absolute Value(x=w171) -> (abs(x)=w153:dbl)
        n71 = Absolute Value(x=w173) -> (abs(x)=w151:dbl)
        n72 = Absolute Value(x=w172) -> (abs(x)=w152:dbl)
        n73 = Absolute Value(x=w170) -> (abs(x)=w154:dbl)
        n74 = Compound Arithmetic op=ADD(w154, w153, w152, w151) -> (w169:dbl)
        n75 = call "SwerveDrive2.0.vi"("Right Trigger"=w187, "RCW"=0.0, "STR"=w167, "FWD"=w145, "Gyro"=w158) -> ()  [unwired: 7 in]
        n76 = Divide(x=w169, y=4.0) -> (x/y=w164:dbl)
        n77 = Multiply(x=4.0 ("y"), y=3.141592653589793) -> (x*y=w155:dbl)
        n78 = Divide(x=w164, y=w155) -> (x/y=w163:dbl)
        n79 = Multiply(x=w163, y=18.0) -> (x*y=w150:dbl)
        n80 = Subtract(x=w165, y=w150) -> (x-y=w147:dbl)
        n81 = Less?(x=w147, y=1.0) -> (x < y?=w148:bool)
        n82 = case shown="True" w148 {
          tunnel: [FALSE ("ignore previous (F)") TRUE ("ignore previous (F)")] -> w144
          frame False {
          }
          frame True {
          }
        }
      }
      frame "Drive to Angle(Distance)" {
        # "Corrects for turning distance"
        # "Wheel Rotations per degree turned"
        # "Wheel diameter"
        n83 = Index Array(array=w196) -> (element #1=w195:dbl, element #2=w194:dbl, element #3=w193:dbl, element #4=w192:dbl)  [unwired: 4 in]
        n84 = call <vilib>:"ADIS16470 RefNum Registry Get.vi"("refnum name"="Gyro") -> ("error out"=w240:errorcluster, "ADIS16470DevRef out"=w239:T9)  [unwired: 9 in]
        n85 = call <vilib>:"ADIS16470 Read.vi"("error in (no error)"=w240, "ADIS16470DevRef"=w239) -> ("ADIS16470 Value"=w238:T19)  [unwired: 6 in, 3 out]
        n86 = call <vilib>:"WPI_MotorControlRefNum Registry Get.vi"("refnum name"="W3 Power") -> ("error out"=w261:errorcluster, "MotorControlDevRef"=w260:T20)  [unwired: 9 in]
        n87 = call <vilib>:"WPI_MotorControlRefNum Registry Get.vi"("refnum name"="W2 Power") -> ("error out"=w263:errorcluster, "MotorControlDevRef"=w262:T20)  [unwired: 9 in]
        n88 = call <vilib>:"WPI_MotorControlRefNum Registry Get.vi"("refnum name"="W4 Power") -> ("error out"=w259:errorcluster, "MotorControlDevRef"=w258:T20)  [unwired: 9 in]
        n89 = call <vilib>:"WPI_MotorControlRefNum Registry Get.vi"("refnum name"="W1 Power") -> ("error out"=w265:errorcluster, "MotorControlDevRef"=w264:T20)  [unwired: 9 in]
        n90 = Unbundle By Name(w238) -> ("ZAngle"=w216:dbl)
        n91 = Subtract(x=w267, y=180.0) -> (x-y=w230:dbl)
        n92 = call <vilib>:"Spark MAX Get Sensor Position.vi"("error in (no error)"=w265, "MotorControlDevRef in"=w264) -> ("Sensor Position"=w250:dbl)  [unwired: 6 in, 3 out]
        n93 = call <vilib>:"Spark MAX Get Sensor Position.vi"("error in (no error)"=w263, "MotorControlDevRef in"=w262) -> ("Sensor Position"=w251:dbl)  [unwired: 6 in, 3 out]
        n94 = call <vilib>:"Spark MAX Get Sensor Position.vi"("error in (no error)"=w261, "MotorControlDevRef in"=w260) -> ("Sensor Position"=w252:dbl)  [unwired: 6 in, 3 out]
        n95 = call <vilib>:"Spark MAX Get Sensor Position.vi"("error in (no error)"=w259, "MotorControlDevRef in"=w258) -> ("Sensor Position"=w253:dbl)  [unwired: 6 in, 3 out]
        n96 = Negate(x=w268) -> (-x=w208:dbl)
        n97 = Subtract(x=w252, y=w193) -> (x-y=w198:dbl)
        n98 = Subtract(x=w251, y=w194) -> (x-y=w199:dbl)
        n99 = Subtract(x=w253, y=w192) -> (x-y=w197:dbl)
        n100 = Subtract(x=w250, y=w195) -> (x-y=w200:dbl)
        n101 = call "Difference.vi"("Angle"=w230, "Gyro"=w216) -> ("Difference"=w231:dbl)  [unwired: 9 in]
        n102 = Subtract(x=w217, y=w216) -> (x-y=w218:dbl)
        n103 = Absolute Value(x=w199) -> (abs(x)=w225:dbl)
        n104 = Absolute Value(x=w198) -> (abs(x)=w224:dbl)
        n105 = Absolute Value(x=w197) -> (abs(x)=w223:dbl)
        n106 = Absolute Value(x=w200) -> (abs(x)=w226:dbl)
        n107 = Negate(x=w218) -> (-x=w243:dbl)
        n108 = Compound Arithmetic op=ADD(w226, w225, w224, w223) -> (w249:dbl)
        n109 = Multiply(x=0.26666, y=w243) -> (x*y=w241:dbl)
        n110 = Divide(x=w249, y=4.0) -> (x/y=w247:dbl)
        n111 = call-poly <vilib>:"PID.vi"("output range"=cluster{"output high":dbl, "output low":dbl} {"output high"=1.0, "output low"=-1.0}, "PID gains"="Drive to Angle(Distance)", "process variable"=w231, "setpoint"=0.0) -> ("output"=w207:dbl)  [unwired: 6 in, 1 out]
        n112 = Multiply(x=4.0 ("y"), y=3.141592653589793) -> (x*y=w236:dbl)
        n113 = Divide(x=w247, y=w236) -> (x/y=w244:dbl)
        n114 = Absolute Value(x=w241) -> (abs(x)=w222:dbl)
        n115 = Absolute Value(x=w244) -> (abs(x)=w227:dbl)
        n116 = Multiply(x=w227, y=18.0) -> (x*y=w219:dbl)
        n117 = Absolute Value(x=w231) -> (abs(x)=w233:dbl)
        n118 = Subtract(x=w219, y=w222) -> (x-y=w220:dbl)
        n119 = Absolute Value(x=w220) -> (abs(x)=w201:dbl)
        n120 = Less?(x=w233, y=2.0) -> (x < y?=w232:bool)
        n121 = Subtract(x=w221, y=w201) -> (x-y=w191:dbl)
        n122 = call-poly <vilib>:"PID.vi"("output range"=cluster{"output high":dbl, "output low":dbl} {"output high"=1.0, "output low"=-1.0}, "PID gains"="Drive to Angle(Distance)", "process variable"=w191, "setpoint"=0.0) -> ("output"=w204:dbl)  [unwired: 6 in, 1 out]
        n123 = Absolute Value(x=w191) -> (abs(x)=w190:dbl)
        n124 = Less?(x=w190, y=7.0) -> (x < y?=w210:bool)
        n125 = Multiply(x=w208, y=w204) -> (x*y=w209:dbl)
        n126 = Compound Arithmetic op=AND(w210, w232) -> (w245:bool)
        n127 = global write "Robot Global Data.vi" "LED STATE"(enum16{"NORMAL", "RAINBOW"}."NORMAL" ("LED STATE")) -> ()
        n128 = Multiply(x=w205, y=w204) -> (x*y=w206:dbl)
        n129 = case shown="True" w245 {
          tunnel: [FALSE ("ignore previous (F)") TRUE ("ignore previous (F)")] -> w203
          frame False {
          }
          frame True {
          }
        }
        n130 = call "SwerveDrive2.0.vi"("Right Trigger"=w269, "RCW"=w207, "STR"=w206, "FWD"=w209, "Gyro"=w216) -> ()  [unwired: 7 in]
      }
      frame "Stop" {
        n131 = call <vilib>:"WPI_MotorControlRefNum Registry Get.vi"("refnum name"="W3 Power") -> ("error out"=w296:errorcluster, "MotorControlDevRef"=w295:T20)  [unwired: 9 in]
        n132 = call <vilib>:"WPI_MotorControlRefNum Registry Get.vi"("refnum name"="W2 Power") -> ("MotorControlDevRef"=w297:T20)  [unwired: 9 in, 1 out]
        n133 = call <vilib>:"WPI_MotorControlRefNum Registry Get.vi"("refnum name"="W4 Power") -> ("error out"=w294:errorcluster, "MotorControlDevRef"=w293:T20)  [unwired: 9 in]
        n134 = call <vilib>:"WPI_MotorControlRefNum Registry Get.vi"("refnum name"="W1 Power") -> ("error out"=w301:errorcluster, "MotorControlDevRef"=w300:T20)  [unwired: 9 in]
        n135 = call <vilib>:"WPI_MotorControlRefNum Registry Get.vi"("refnum name"="W3 Rotation") -> ("error out"=w281:errorcluster, "MotorControlDevRef"=w280:T20)  [unwired: 9 in]
        n136 = call <vilib>:"WPI_MotorControlRefNum Registry Get.vi"("refnum name"="W2 Rotation") -> ("MotorControlDevRef"=w282:T20)  [unwired: 9 in, 1 out]
        n137 = call <vilib>:"WPI_MotorControlRefNum Registry Get.vi"("refnum name"="W4 Rotation") -> ("error out"=w279:errorcluster, "MotorControlDevRef"=w278:T20)  [unwired: 9 in]
        n138 = call <vilib>:"WPI_MotorControlRefNum Registry Get.vi"("refnum name"="W1 Rotation") -> ("error out"=w286:errorcluster, "MotorControlDevRef"=w285:T20)  [unwired: 9 in]
        n139 = call <vilib>:"WPI_MotorControlSetOutput.vi"("error in (no error)"=w279, "Output"=0.0, "MotorControlDevRef"=w278) -> ()  [unwired: 6 in, 3 out]
        n140 = call <vilib>:"WPI_MotorControlSetOutput.vi"("error in (no error)"=w281, "Output"=0.0, "MotorControlDevRef"=w280) -> ()  [unwired: 6 in, 3 out]
        n141 = call <vilib>:"WPI_MotorControlSetOutput.vi"("error in (no error)"=w294, "Output"=0.0, "MotorControlDevRef"=w293) -> ()  [unwired: 6 in, 3 out]
        n142 = call <vilib>:"WPI_MotorControlSetOutput.vi"("error in (no error)"=w286, "Output"=0.0, "MotorControlDevRef"=w285) -> ()  [unwired: 6 in, 3 out]
        n143 = call <vilib>:"WPI_MotorControlSetOutput.vi"("Output"=0.0, "MotorControlDevRef"=w282) -> ()  [unwired: 7 in, 3 out]
        n144 = call <vilib>:"WPI_MotorControlSetOutput.vi"("error in (no error)"=w296, "Output"=0.0, "MotorControlDevRef"=w295) -> ()  [unwired: 6 in, 3 out]
        n145 = call <vilib>:"WPI_MotorControlSetOutput.vi"("error in (no error)"=w301, "Output"=0.0, "MotorControlDevRef"=w300) -> ()  [unwired: 6 in, 3 out]
        n146 = call <vilib>:"WPI_MotorControlSetOutput.vi"("Output"=0.0, "MotorControlDevRef"=w297) -> ()  [unwired: 7 in, 3 out]
      }
      frame "Balance" {
        n147 = call <vilib>:"ADIS16470 RefNum Registry Get.vi"("refnum name"="Gyro") -> ("error out"=w323:errorcluster, "ADIS16470DevRef out"=w322:T9)  [unwired: 9 in]
        n148 = call <vilib>:"ADIS16470 Read.vi"("error in (no error)"=w323, "ADIS16470DevRef"=w322) -> ("ADIS16470 Value"=w321:T19)  [unwired: 6 in, 3 out]
        n149 = Unbundle By Name(w321) -> ("ZAngle"=w317:dbl, "XAngle"=w309:dbl)
        n150 = call-poly <vilib>:"PID.vi"("output range"=cluster{"output high":dbl, "output low":dbl} {"output high"=0.5, "output low"=-0.5}, "PID gains"="Balance", "process variable"=w309, "setpoint"=0.0) -> ("output"=w308:dbl)  [unwired: 6 in, 1 out]
        n151 = Negate(x=w308) -> (-x=w307:dbl)
        n152 = call "SwerveDrive2.0.vi"("Right Trigger"=0.0, "RCW"=0.0, "STR"=0.0, "FWD"=w307, "Gyro"=w317) -> ()  [unwired: 7 in]
        n153 = Absolute Value(x=w309) -> (abs(x)=w313:dbl)
        n154 = Less?(x=w313, y=1.0) -> (x < y?=w306:bool)
        n155 = case shown="False" w306 {
          frame False {
            n156 = global write "Robot Global Data.vi" "LED STATE"(enum16{"NORMAL", "RAINBOW"}."NORMAL" ("LED STATE")) -> ()
          }
          frame True {
            n157 = global write "Robot Global Data.vi" "LED STATE"(enum16{"NORMAL", "RAINBOW"}."RAINBOW" ("LED STATE")) -> ()
          }
        }
      }
      frame "Look At Cone" {
        n158 = flat-sequence {
          tunnel: [w333] -> w326
          frame #0 {
            n159 = global write "Robot Global Data.vi" "target"(T8."Cone" ("target")) -> ()
          }
          frame #1 {
            n160 = call <vilib>:"ADIS16470 RefNum Registry Get.vi"("refnum name"="Gyro") -> ("error out"=w336:errorcluster, "ADIS16470DevRef out"=w337:T9)  [unwired: 9 in]
            n161 = global read "Robot Global Data.vi" "VisionAngle"() -> (w329:dbl)
            n162 = call <vilib>:"ADIS16470 Read.vi"("error in (no error)"=w336, "ADIS16470DevRef"=w337) -> ("ADIS16470 Value"=w338:T19)  [unwired: 6 in, 3 out]
            n163 = Unbundle By Name(w338) -> ("ZAngle"=w339:dbl)
            n164 = Absolute Value(x=w329) -> (abs(x)=w330:dbl)
            n165 = Greater?(x=w330, y=20.0) -> (0:w331:bool)
            n166 = case shown="True" w331 {
              tunnel: w339 -> [_ w347]
              tunnel: w329 -> [_ w341]
              frame False {
              }
              frame True {
                (unwired) 160.0 ("x")
                n167 = call-poly <vilib>:"PID.vi"("output range"=cluster{"output high":dbl, "output low":dbl} {"output high"=0.1, "output low"=-0.1}, "PID gains"="Look At Cone", "process variable"=w341, "setpoint"=0.0) -> ("output"=w348:dbl)  [unwired: 6 in, 1 out]
                n168 = Negate(x=w348) -> (-x=w350:dbl)
                n169 = call "SwerveDrive2.0.vi"("Right Trigger"=0.0, "RCW"=w350, "STR"=0.0, "FWD"=0.0, "Gyro"=w347) -> ()  [unwired: 7 in]
              }
            }
            n170 = Absolute Value(x=w329) -> (abs(x)=w340:dbl)
            n171 = Less?(x=w340, y=20.0) -> (x < y?=w333:bool)
          }
        }
      }
      frame "Look At Cube" {
        n172 = flat-sequence {
          tunnel: [w358] -> w351
          frame #0 {
            n173 = global write "Robot Global Data.vi" "target"(T8."Cube" ("target")) -> ()
          }
          frame #1 {
            n174 = global read "Robot Global Data.vi" "VisionAngle"() -> (w357:dbl)
            n175 = call <vilib>:"ADIS16470 RefNum Registry Get.vi"("refnum name"="Gyro") -> ("error out"=w361:errorcluster, "ADIS16470DevRef out"=w362:T9)  [unwired: 9 in]
            n176 = call <vilib>:"ADIS16470 Read.vi"("error in (no error)"=w361, "ADIS16470DevRef"=w362) -> ("ADIS16470 Value"=w363:T19)  [unwired: 6 in, 3 out]
            n177 = Absolute Value(x=w357) -> (abs(x)=w356:dbl)
            n178 = Unbundle By Name(w363) -> ("ZAngle"=w364:dbl)
            n179 = Greater?(x=w356, y=15.0) -> (0:w354:bool)
            n180 = case shown="True" w354 {
              tunnel: w357 -> [_ w376]
              tunnel: w364 -> [_ w372]
              frame False {
                n181 = call "Swerve.vi"("SubSystem Data"=T2 {"Operation"=enum."Stop", "Gyro"=0.0, "FWD"=0.0, "STR"=0.0, "X rotate"=0.0, "Y rotate"=0.0, "Time"=0.0, "Distance"=0.0, "Right Trigger"=0.0, "Angle"=0.0, "Start Angle"=0.0, "Tag ID"=0.0, "Start Positions"=[]}) -> ()  [unwired: 10 in, 1 out]
              }
              frame True {
                n182 = call-poly <vilib>:"PID.vi"("output range"=cluster{"output high":dbl, "output low":dbl} {"output high"=0.5, "output low"=-0.5}, "PID gains"="Look At Cube", "process variable"=w376, "setpoint"=0.0) -> ("output"=w373:dbl)  [unwired: 6 in, 1 out]
                n183 = Negate(x=w373) -> (-x=w375:dbl)
                n184 = call "SwerveDrive2.0.vi"("Right Trigger"=0.0, "RCW"=w375, "STR"=0.0, "FWD"=0.0, "Gyro"=w372) -> ()  [unwired: 7 in]
              }
            }
            n185 = Absolute Value(x=w357) -> (abs(x)=w365:dbl)
            n186 = Less?(x=w365, y=15.0) -> (x < y?=w358:bool)
          }
        }
      }
      frame "Move To Tag" {
        n187 = flat-sequence {
          tunnel: w380 -> [w382]
          tunnel: [w382] -> w377
          tunnel: [w383] -> w379
          tunnel: w377 -> [w386]
          frame #0 {
            n188 = global write "Robot Global Data.vi" "target"(T8."AprilTag" ("target")) -> ()
          }
          frame #1 {
            n189 = global read "Robot Global Data.vi" "Detected Tags"() -> (w387:T24)
            n190 = for {
              tunnel: w387 -> [w397] mode=indexing
              tunnel: w386 -> [w395]
              tunnel: [w392] -> w385 mode=indexing
              n191 = Unbundle By Name(w397) -> ("Center.X"=w394:dbl, "tag ID"=w396:i32)
              n192 = Equal?(x=w396, y=w395) -> (x = y?=w393:bool)
              n193 = case shown="True" w393 {
                tunnel: w394 -> [_ w411]
                tunnel: [0.0 w399] -> w392
                frame False {
                }
                frame True {
                  n194 = Subtract(x=w411, y=160.0 ("x")) -> (x-y=w399:dbl)
                  n195 = call-poly <vilib>:"PID.vi"("output range"=cluster{"output high":dbl, "output low":dbl} {"output high"=0.1, "output low"=-0.1}, "PID gains"="AprilTag", "process variable"=w399, "setpoint"=0.0) -> ("output"=w413:dbl)  [unwired: 6 in, 1 out]
                  n196 = call <vilib>:"ADIS16470 RefNum Registry Get.vi"("refnum name"="Gyro") -> ("error out"=w406:errorcluster, "ADIS16470DevRef out"=w407:T9)  [unwired: 9 in]
                  n197 = call <vilib>:"ADIS16470 Read.vi"("error in (no error)"=w406, "ADIS16470DevRef"=w407) -> ("ADIS16470 Value"=w408:T19)  [unwired: 6 in, 3 out]
                  n198 = Unbundle By Name(w408) -> ("ZAngle"=w404:dbl)
                  n199 = call "SwerveDrive2.0.vi"("Right Trigger"=0.0, "RCW"=0.0, "STR"=w413, "FWD"=0.0, "Gyro"=w404) -> ()  [unwired: 7 in]
                }
              }
            }
            n200 = for {
              tunnel: [w391] -> w384 mode=indexing
              tunnel: w385 -> [w390] mode=indexing
              n201 = Absolute Value(x=w390) -> (abs(x)=w389:dbl)
              n202 = Less?(x=w389, y=10.0) -> (x < y?=w391:bool)
            }
            n203 = And Array Elements(Boolean array=w384) -> (logical AND=w383:bool)
          }
        }
      }
      frame "Move To Tape" {
        n204 = flat-sequence {
          tunnel: [w417] -> w415
          frame #0 {
            n205 = global write "Robot Global Data.vi" "target"(T8."Reflective Tape" ("target")) -> ()
          }
          frame #1 {
            n206 = global read "Robot Global Data.vi" "VisionAngle"() -> (w420:dbl)
            n207 = call <vilib>:"ADIS16470 RefNum Registry Get.vi"("refnum name"="Gyro") -> ("error out"=w427:errorcluster, "ADIS16470DevRef out"=w428:T9)  [unwired: 9 in]
            n208 = call <vilib>:"ADIS16470 Read.vi"("error in (no error)"=w427, "ADIS16470DevRef"=w428) -> ("ADIS16470 Value"=w429:T19)  [unwired: 6 in, 3 out]
            n209 = Unbundle By Name(w429) -> ("ZAngle"=w425:dbl)
            n210 = call-poly <vilib>:"PID.vi"("output range"=cluster{"output high":dbl, "output low":dbl} {"output high"=0.1, "output low"=-0.1}, "PID gains"="Tape", "process variable"=w420, "setpoint"=0.0) -> ("output"=w432:dbl)  [unwired: 6 in, 1 out]
            n211 = Absolute Value(x=w420) -> (abs(x)=w419:dbl)
            n212 = Less?(x=w419, y=10.0) -> (x < y?=w417:bool)
            n213 = call "SwerveDrive2.0.vi"("Right Trigger"=0.0, "RCW"=0.0, "STR"=w432, "FWD"=0.0, "Gyro"=w425) -> ()  [unwired: 7 in]
          }
        }
      }
    }
    n214 = call "Swerve Check for New Command.vi"("Current Command"=w18, "Wait time (ms)"=w23, "Finished?"=w6) -> ("Completion"=w19:T4, "Subsystem Name"=w20:string, "Current Command"=w21:T2, "Initial Trace String"=w22:string, "NextCommand"=w24:T7)  [unwired: 4 in]
    n215 = case shown="\"Successful\", \"Aborted\"" w19 {
      selector: w19 -> [_ w440]
      tunnel: w22 -> [_ w436]
      tunnel: w21 -> [_ w437]
      tunnel: w20 -> [_ w433]
      frame "Incomplete", Default {
        # "Continuing current command"
      }
      frame "Successful", "Aborted" {
        # "Report and setup for next command"
        n216 = Unbundle By Name(w437) -> ("Gyro"=w439:dbl, "Y rotate"=w434:dbl)
        n217 = Format Into String(format string="S %.1f, D %f", initial string=w436, w439, w434) -> (resulting string=w435:string)  [unwired: 1 in, 1 out]
        "Current\nCmd" <- w435
        n218 = call <vilib>:"Trace Results.vi"("Status of previous command"=w440, "Description"=w435, "Subsystem"=w433) -> ()  [unwired: 9 in]
      }
    }
    n219 = disable-structure shown="Disabled" {
      frame Disabled {
        # "Publish"
        n220 = call-poly <vilib>:"NT Write Value.vi"() -> ()  [unwired: 11 in, 1 out]
      }
      frame Enabled {
      }
    }
  }
  n221 = while {
    tunnel: w1 -> [w447]
    stop <- FALSE stop-if-true
    n222 = call "Swerve Controller Interactive Check.vi"("Interactive Command in"="Interactive Values", "Default Command"=w447, "Buttons"="Buttons") -> ("Interactive Command out"=w444:T2, "Trace String"=w445:string, "Schedule"=w446:bool)  [unwired: 6 in]
    n223 = case shown="True" w446 {
      tunnel: [w458 w463] -> w443
      tunnel: w444 -> [_ w461]
      tunnel: [w454 w459] -> w442
      tunnel: w445 -> [_ w462]
      frame False {
        n224 = Tick Count (ms)() -> (millisecond timer value=w453:u32)
        n225 = call "Read Swerve Operation.vi"() -> ("Command Info"=w451:T5, "SubSystem Data"=w452:T2)  [unwired: 9 in, 1 out]
        n226 = Unbundle(w452) -> ("Operation"=w457:T3, "Gyro"=w455:dbl)  [unwired: 11 out]
        n227 = Unbundle(w451) -> ("Status"=w458:T4)  [unwired: 2 out]
        n228 = Subtract(x=w453, y=w457) -> (x-y=w456:u32)
        n229 = Bundle(w456, "Gyro"=w455) -> (w454:cluster{u32, "Gyro":dbl})  [unwired: 1 in]
      }
      frame True {
        n230 = call "Swerve Command Helper.vi"("Description"=w462, "SubSystem Data"=w461) -> ("Command Info Out"=w460:T5, "Command Timing"=w459:cluster{"Start Time (ms)":u32, "Iterations":i32})  [unwired: 7 in, 1 out]
        n231 = Unbundle(w460) -> ("Status"=w463:T4)  [unwired: 2 out]
      }
    }
    "Status" <- w443
    "Command Timing" <- w442
    n232 = Wait (ms)(milliseconds to wait=u32 20) -> ()  [unwired: 1 out]
  }
